vi "ms2hhmmss.vi"(1 "ms":u64) -> (0 "hh:mm:ss":string)   [LabVIEW 2019]
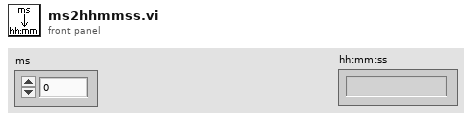
[diagram p1: front panel]
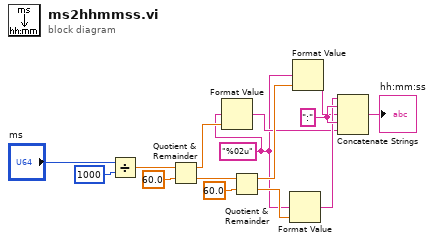
[diagram p0: block diagram]
diagram:
  w2 = "%02u" ("format string")
  w10 = ":" ("string")
  n1 = Divide(x="ms", y=u32 1000) -> (x/y=w14:dbl)
  n2 = Quotient & Remainder(x=w14, y=60.0) -> (x-y*floor(x/y)=w4:dbl, floor(x/y)=w11:dbl)
  n3 = Format Value(format string=w2, value (0)=w4) -> (output string=w3:string)  [unwired: 1 in]
  n4 = Quotient & Remainder(x=w11, y=60.0) -> (x-y*floor(x/y)=w5:dbl, floor(x/y)=w8:dbl)
  n5 = Format Value(format string=w2, value (0)=w8) -> (output string=w7:string)  [unwired: 1 in]
  n6 = Format Value(format string=w2, value (0)=w5) -> (output string=w6:string)  [unwired: 1 in]
  n7 = Concatenate Strings(w7, w10, w6, w10, w3) -> (→"hh:mm:ss":string)
